vi "InGaAs-GaAs QDSL-111221a.vi"() -> ()   [LabVIEW 2011]
panel:
  out "step number  5":i32
  in  "Number of \nGrowth Steps 5":i32=10
  out "step number  4":i32
  in  "Number of \nGrowth Steps 4":i32=10
  out "step number  3":i32
  in  "Number of \nGrowth Steps 3":i32=10
  out "step number  2":i32
  in  "Number of \nGrowth Steps 2":i32=10
  in  "Indium Flow 2":dbl=55.0
  in  "Ga Flow 3":dbl=2.0
  in  "Ga Flow 2":dbl=2.41
  in  "Ga Flow 1":dbl=5.49
  in  "Indium Flow":dbl=44.0
  in  "Number of \nGrowth Steps":i32=10
  out "step number":i32
  in  "As_Gas Flow":dbl=3.4
  in  "Manifold H2 Flow":dbl=720.0
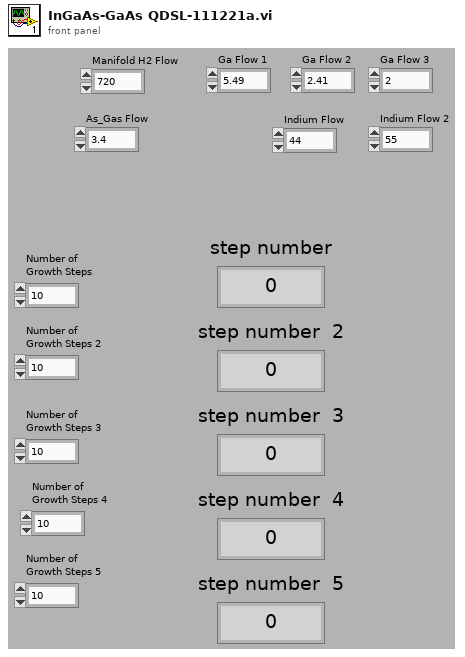
[diagram p1: front panel]
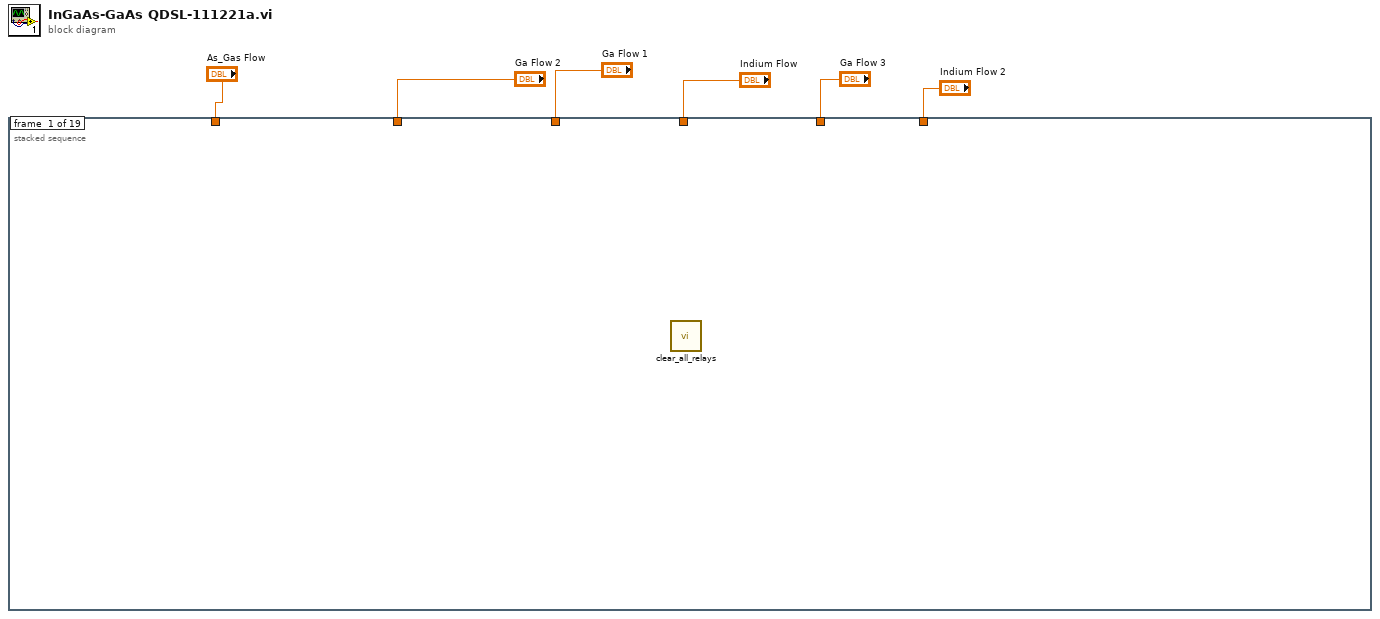
[diagram p0: block diagram]
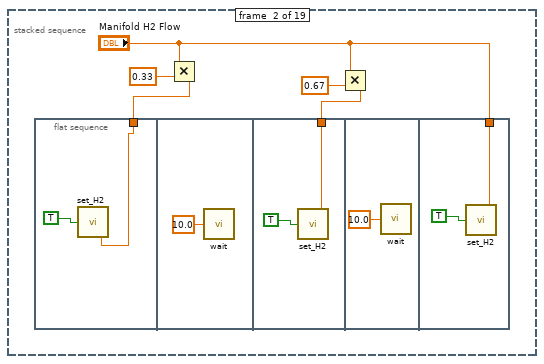
[diagram p2: hidden frame]
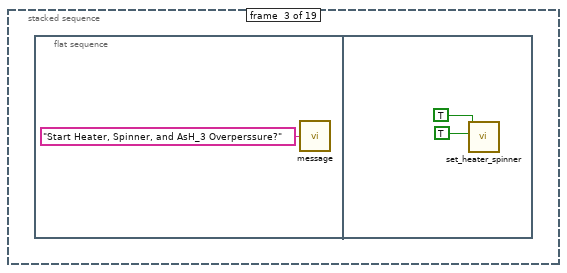
[diagram p3: hidden frame]
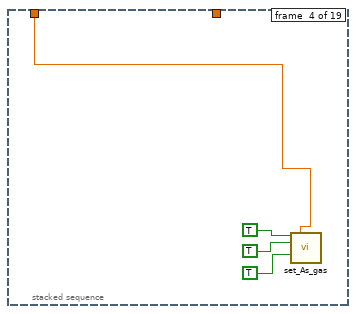
[diagram p4: hidden frame]
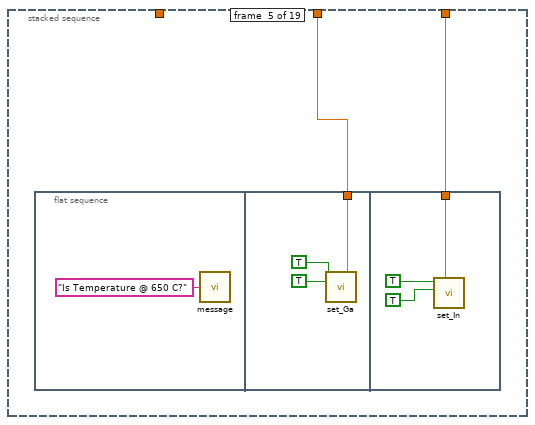
[diagram p5: hidden frame]
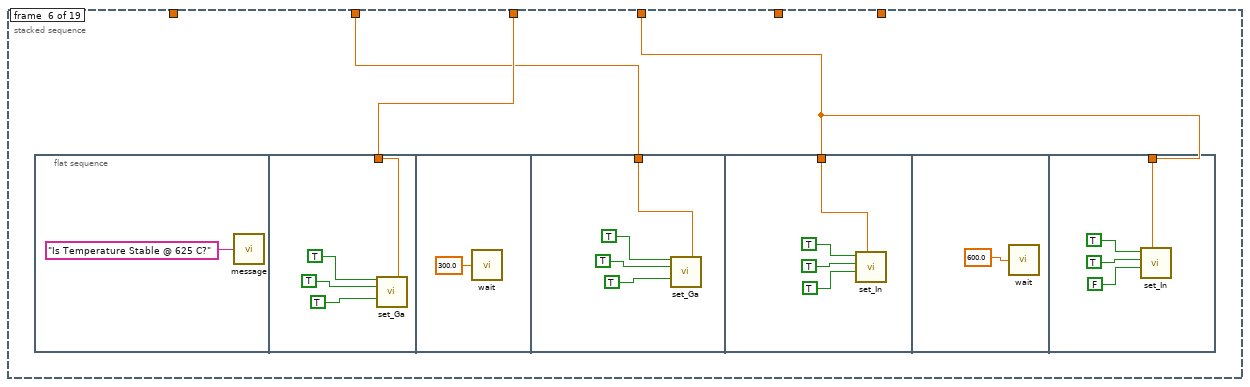
[diagram p6: hidden frame]
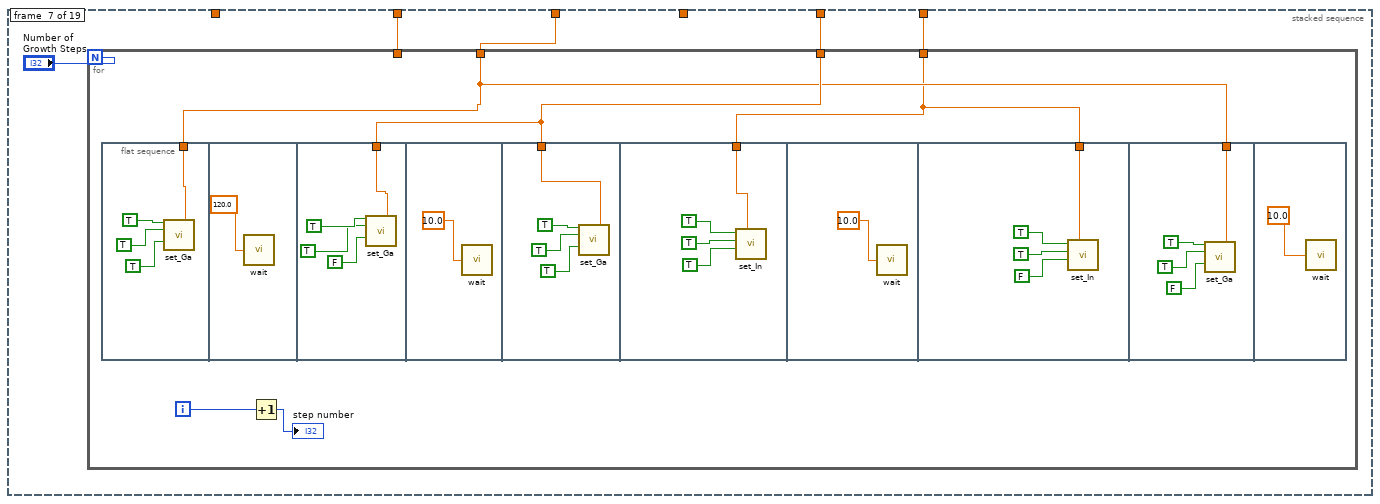
[diagram p7: hidden frame]
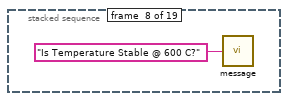
[diagram p8: hidden frame]
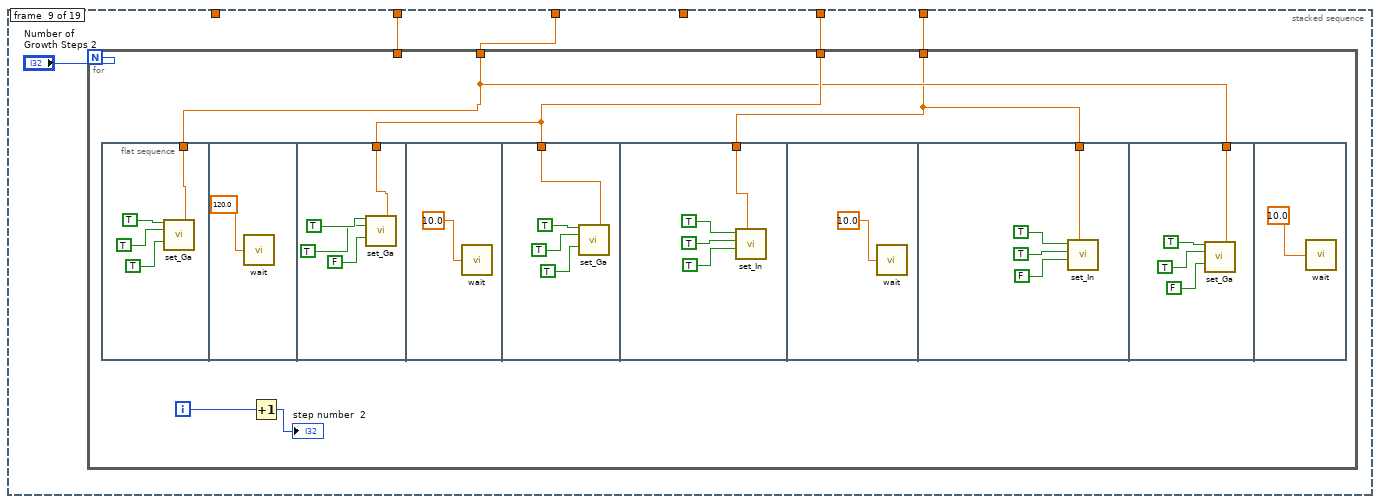
[diagram p9: hidden frame]
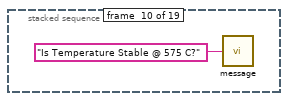
[diagram p10: hidden frame]
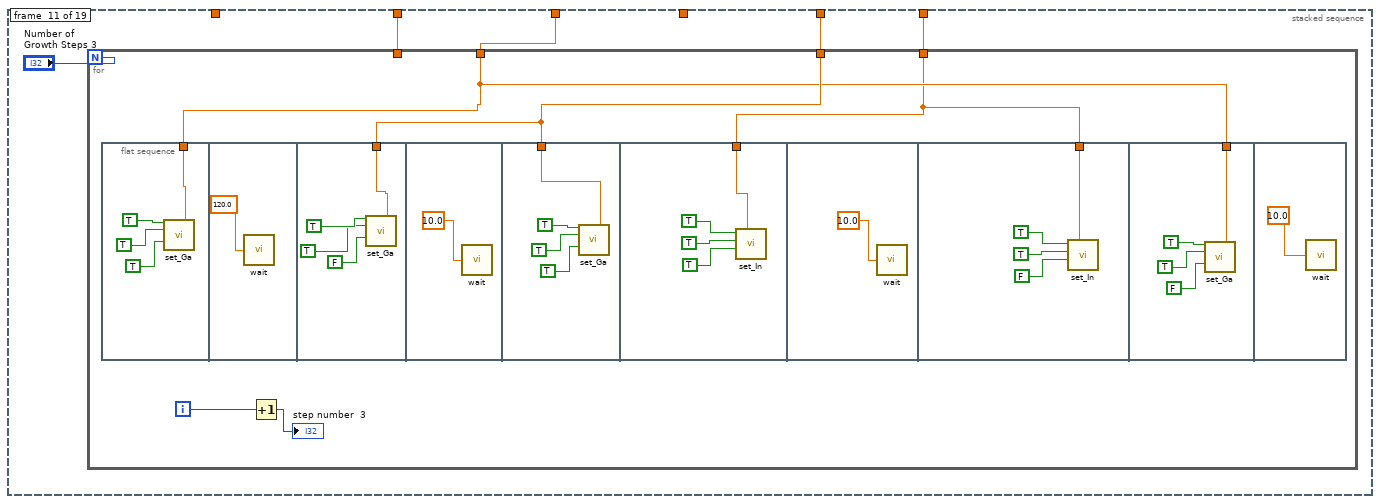
[diagram p11: hidden frame]
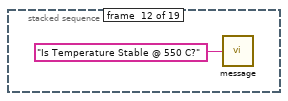
[diagram p12: hidden frame]
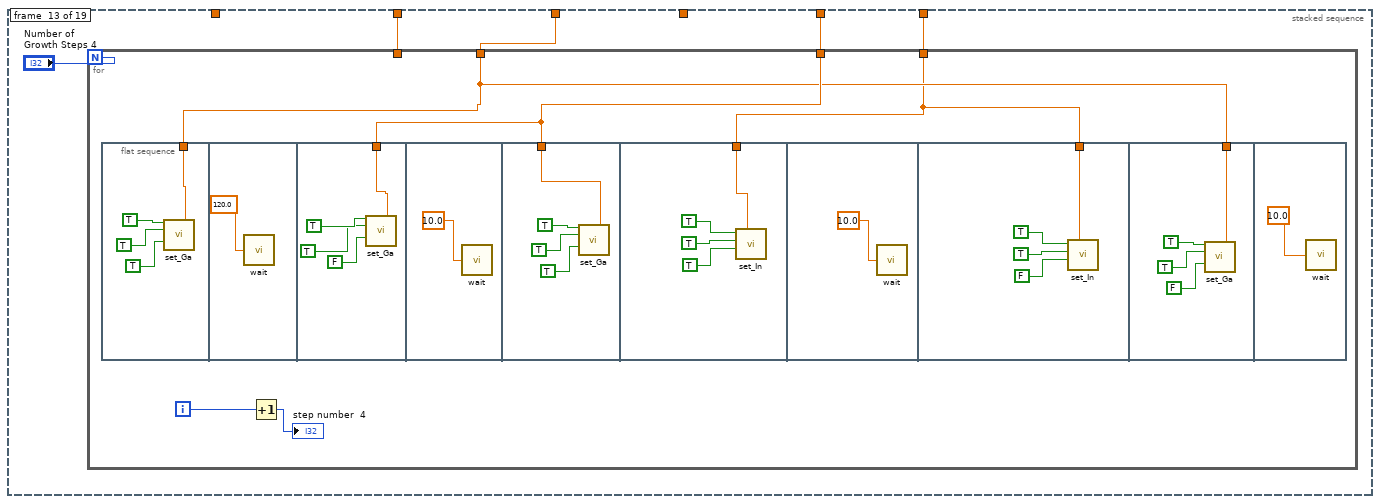
[diagram p13: hidden frame]
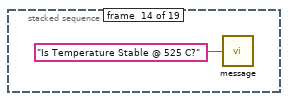
[diagram p14: hidden frame]
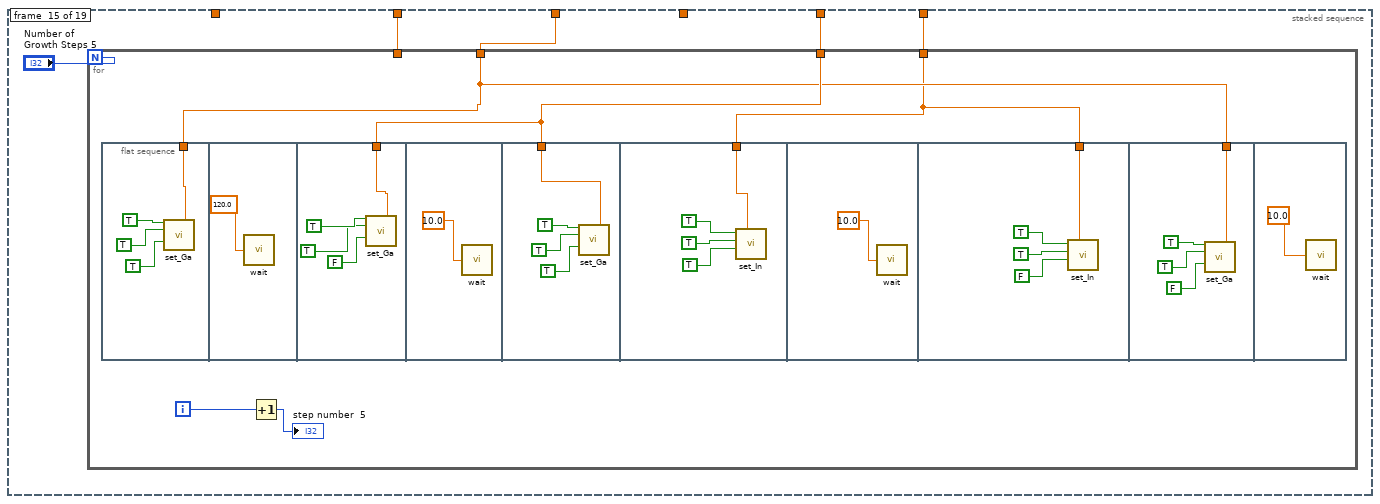
[diagram p15: hidden frame]
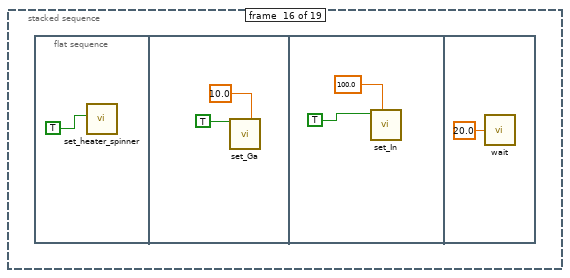
[diagram p16: hidden frame]
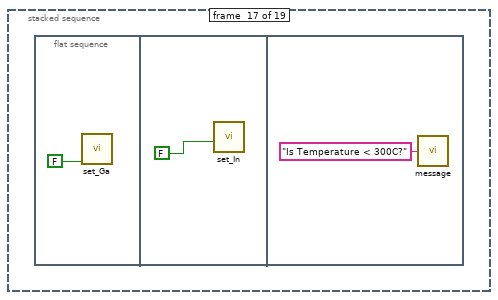
[diagram p17: hidden frame]
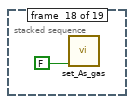
[diagram p18: hidden frame]
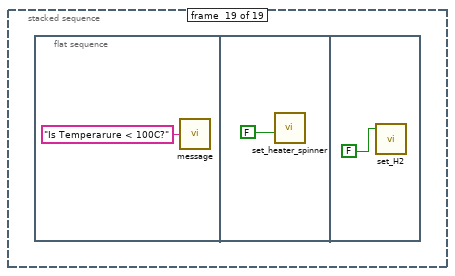
[diagram p19: hidden frame]
diagram:
  n1 = stacked-sequence {
    tunnel: "Ga Flow 1" -> [_ _ _ _ w28 w38 w61 _ w100 _ w139 _ w178 _ w217 _ _ _ _]
    tunnel: "As_Gas Flow" -> [_ _ _ w23 _ _ _ _ _ _ _ _ _ _ _ _ _ _ _]
    tunnel: "Indium Flow" -> [_ _ _ _ w27 w36 _ _ _ _ _ _ _ _ _ _ _ _ _]
    tunnel: "Ga Flow 2" -> [_ _ _ _ _ w37 w60 _ w99 _ w138 _ w177 _ w216 _ _ _ _]
    tunnel: "Ga Flow 3" -> [_ _ _ _ _ _ w59 _ w98 _ w137 _ w176 _ w215 _ _ _ _]
    tunnel: "Indium Flow 2" -> [_ _ _ _ _ _ w58 _ w97 _ w136 _ w175 _ w214 _ _ _ _]
    frame #0 {
      n2 = call "clear_all_relays.vi"() -> ()  [unwired: 2 out]
    }
    frame #1 {
      n3 = flat-sequence {
        tunnel: w11 -> [w12]
        tunnel: w9 -> [w15]
        tunnel: "Manifold H2 Flow" -> [w18]
        frame #0 {
          n4 = call "set_H2.vi"("Manifold H2 Flow"=w12, "H2 Active"=TRUE) -> ()  [unwired: 2 in, 2 out]
        }
        frame #1 {
          n5 = call "wait.vi"("Wait (s)"=10.0) -> ()
        }
        frame #2 {
          n6 = call "set_H2.vi"("Manifold H2 Flow"=w15, "H2 Active"=TRUE) -> ()  [unwired: 2 in, 2 out]
        }
        frame #3 {
          n7 = call "wait.vi"("Wait (s)"=10.0) -> ()
        }
        frame #4 {
          n8 = call "set_H2.vi"("Manifold H2 Flow"=w18, "H2 Active"=TRUE) -> ()  [unwired: 2 in, 2 out]
        }
      }
      n9 = Multiply(x="Manifold H2 Flow", y=0.33) -> (x*y=w11:dbl)
      n10 = Multiply(x="Manifold H2 Flow", y=0.67) -> (x*y=w9:dbl)
    }
    frame #2 {
      n11 = flat-sequence {
        frame #0 {
          n12 = call "message.vi"("message"="Start Heater, Spinner, and AsH_3 Overperssure?") -> ()
        }
        frame #1 {
          n13 = call "set_heater_spinner.vi"("Spinner"=TRUE, "Heater"=TRUE) -> ()  [unwired: 1 in, 7 out]
        }
      }
    }
    frame #3 {
      n14 = call "set_As_gas.vi"("As_Gas Active"=TRUE, "As_Gas Flow"=w23, "As_Gas In"=TRUE, "As_Gas Run"=TRUE) -> ()  [unwired: 2 in, 10 out]
    }
    frame #4 {
      n15 = flat-sequence {
        tunnel: w28 -> [w30]
        tunnel: w27 -> [w33]
        frame #0 {
          n16 = call "message.vi"("message"="Is Temperature @ 650 C?") -> ()
        }
        frame #1 {
          n17 = call "set_Ga.vi"("Ga Active"=TRUE, "Ga Flow 1"=w30, "Ga Bubbler"=TRUE) -> ()  [unwired: 5 in, 8 out]
        }
        frame #2 {
          n18 = call "set_In.vi"("Indium Flow"=w33, "In Bubbler"=TRUE ("Ga Bubbler"), "In Active"=TRUE ("Ga Active")) -> ()  [unwired: 2 in, 5 out]
        }
      }
    }
    frame #5 {
      n19 = flat-sequence {
        tunnel: w38 -> [w40]
        tunnel: w37 -> [w45]
        tunnel: w36 -> [w49]
        tunnel: w36 -> [w54]
        frame #0 {
          n20 = call "message.vi"("message"="Is Temperature Stable @ 625 C?") -> ()
        }
        frame #1 {
          n21 = call "set_Ga.vi"("Ga Active"=TRUE ("P_Gas Active"), "Ga Flow 1"=w40, "Ga Bubbler"=TRUE ("P_Gas In"), "Ga Run"=TRUE ("P_Gas Run")) -> ()  [unwired: 4 in, 8 out]
        }
        frame #2 {
          n22 = call "wait.vi"("Wait (s)"=300.0) -> ()
        }
        frame #3 {
          n23 = call "set_Ga.vi"("Ga Active"=TRUE ("P_Gas Active"), "Ga Flow 1"=w45, "Ga Bubbler"=TRUE ("P_Gas In"), "Ga Run"=TRUE ("P_Gas Run")) -> ()  [unwired: 4 in, 8 out]
        }
        frame #4 {
          n24 = call "set_In.vi"("Indium Flow"=w49, "In Run"=TRUE ("P_Gas Run"), "In Bubbler"=TRUE ("P_Gas In"), "In Active"=TRUE ("P_Gas Active")) -> ()  [unwired: 1 in, 5 out]
        }
        frame #5 {
          n25 = call "wait.vi"("Wait (s)"=600.0) -> ()
        }
        frame #6 {
          n26 = call "set_In.vi"("Indium Flow"=w54, "In Run"=FALSE ("P_Gas Run"), "In Bubbler"=TRUE ("P_Gas In"), "In Active"=TRUE ("P_Gas Active")) -> ()  [unwired: 1 in, 5 out]
        }
      }
    }
    frame #6 {
      n27 = for {
        N: "Number of \nGrowth Steps" -> [_]
        tunnel: w61 -> [w64]
        tunnel: w60 -> [_]
        tunnel: w59 -> [w65]
        tunnel: w58 -> [w63]
        i -> [w66]
        n28 = flat-sequence {
          tunnel: w64 -> [w68]
          tunnel: w65 -> [w73]
          tunnel: w65 -> [w78]
          tunnel: w63 -> [w82]
          tunnel: w63 -> [w87]
          tunnel: w64 -> [w91]
          frame #0 {
            n29 = call "set_Ga.vi"("Ga Active"=TRUE ("P_Gas Active"), "Ga Flow 1"=w68, "Ga Bubbler"=TRUE ("P_Gas In"), "Ga Run"=TRUE ("P_Gas Run")) -> ()  [unwired: 4 in, 8 out]
          }
          frame #1 {
            n30 = call "wait.vi"("Wait (s)"=120.0) -> ()
          }
          frame #2 {
            n31 = call "set_Ga.vi"("Ga Active"=TRUE ("P_Gas Active"), "Ga Flow 1"=w73, "Ga Bubbler"=TRUE ("P_Gas In"), "Ga Run"=FALSE ("P_Gas Run")) -> ()  [unwired: 4 in, 8 out]
          }
          frame #3 {
            n32 = call "wait.vi"("Wait (s)"=10.0) -> ()
          }
          frame #4 {
            n33 = call "set_Ga.vi"("Ga Active"=TRUE ("P_Gas Active"), "Ga Flow 1"=w78, "Ga Bubbler"=TRUE ("P_Gas In"), "Ga Run"=TRUE ("P_Gas Run")) -> ()  [unwired: 4 in, 8 out]
          }
          frame #5 {
            n34 = call "set_In.vi"("Indium Flow"=w82, "In Run"=TRUE ("P_Gas Run"), "In Bubbler"=TRUE ("P_Gas In"), "In Active"=TRUE ("P_Gas Active")) -> ()  [unwired: 1 in, 5 out]
          }
          frame #6 {
            n35 = call "wait.vi"("Wait (s)"=10.0) -> ()
          }
          frame #7 {
            n36 = call "set_In.vi"("Indium Flow"=w87, "In Run"=FALSE ("P_Gas Run"), "In Bubbler"=TRUE ("P_Gas In"), "In Active"=TRUE ("P_Gas Active")) -> ()  [unwired: 1 in, 5 out]
          }
          frame #8 {
            n37 = call "set_Ga.vi"("Ga Active"=TRUE ("P_Gas Active"), "Ga Flow 1"=w91, "Ga Bubbler"=TRUE ("P_Gas In"), "Ga Run"=FALSE ("P_Gas Run")) -> ()  [unwired: 4 in, 8 out]
          }
          frame #9 {
            n38 = call "wait.vi"("Wait (s)"=10.0) -> ()
          }
        }
        n39 = Increment(x=w66) -> (x+1=→"step number":i32)
      }
    }
    frame #7 {
      n40 = call "message.vi"("message"="Is Temperature Stable @ 600 C?") -> ()
    }
    frame #8 {
      n41 = for {
        N: "Number of \nGrowth Steps 2" -> [_]
        tunnel: w100 -> [w103]
        tunnel: w99 -> [_]
        tunnel: w98 -> [w104]
        tunnel: w97 -> [w102]
        i -> [w105]
        n42 = flat-sequence {
          tunnel: w103 -> [w107]
          tunnel: w104 -> [w112]
          tunnel: w104 -> [w117]
          tunnel: w102 -> [w121]
          tunnel: w102 -> [w126]
          tunnel: w103 -> [w130]
          frame #0 {
            n43 = call "set_Ga.vi"("Ga Active"=TRUE ("P_Gas Active"), "Ga Flow 1"=w107, "Ga Bubbler"=TRUE ("P_Gas In"), "Ga Run"=TRUE ("P_Gas Run")) -> ()  [unwired: 4 in, 8 out]
          }
          frame #1 {
            n44 = call "wait.vi"("Wait (s)"=120.0) -> ()
          }
          frame #2 {
            n45 = call "set_Ga.vi"("Ga Active"=TRUE ("P_Gas Active"), "Ga Flow 1"=w112, "Ga Bubbler"=TRUE ("P_Gas In"), "Ga Run"=FALSE ("P_Gas Run")) -> ()  [unwired: 4 in, 8 out]
          }
          frame #3 {
            n46 = call "wait.vi"("Wait (s)"=10.0) -> ()
          }
          frame #4 {
            n47 = call "set_Ga.vi"("Ga Active"=TRUE ("P_Gas Active"), "Ga Flow 1"=w117, "Ga Bubbler"=TRUE ("P_Gas In"), "Ga Run"=TRUE ("P_Gas Run")) -> ()  [unwired: 4 in, 8 out]
          }
          frame #5 {
            n48 = call "set_In.vi"("Indium Flow"=w121, "In Run"=TRUE ("P_Gas Run"), "In Bubbler"=TRUE ("P_Gas In"), "In Active"=TRUE ("P_Gas Active")) -> ()  [unwired: 1 in, 5 out]
          }
          frame #6 {
            n49 = call "wait.vi"("Wait (s)"=10.0) -> ()
          }
          frame #7 {
            n50 = call "set_In.vi"("Indium Flow"=w126, "In Run"=FALSE ("P_Gas Run"), "In Bubbler"=TRUE ("P_Gas In"), "In Active"=TRUE ("P_Gas Active")) -> ()  [unwired: 1 in, 5 out]
          }
          frame #8 {
            n51 = call "set_Ga.vi"("Ga Active"=TRUE ("P_Gas Active"), "Ga Flow 1"=w130, "Ga Bubbler"=TRUE ("P_Gas In"), "Ga Run"=FALSE ("P_Gas Run")) -> ()  [unwired: 4 in, 8 out]
          }
          frame #9 {
            n52 = call "wait.vi"("Wait (s)"=10.0) -> ()
          }
        }
        n53 = Increment(x=w105) -> (x+1=→"step number  2":i32)
      }
    }
    frame #9 {
      n54 = call "message.vi"("message"="Is Temperature Stable @ 575 C?") -> ()
    }
    frame #10 {
      n55 = for {
        N: "Number of \nGrowth Steps 3" -> [_]
        tunnel: w139 -> [w142]
        tunnel: w138 -> [_]
        tunnel: w137 -> [w143]
        tunnel: w136 -> [w141]
        i -> [w144]
        n56 = flat-sequence {
          tunnel: w142 -> [w146]
          tunnel: w143 -> [w151]
          tunnel: w143 -> [w156]
          tunnel: w141 -> [w160]
          tunnel: w141 -> [w165]
          tunnel: w142 -> [w169]
          frame #0 {
            n57 = call "set_Ga.vi"("Ga Active"=TRUE ("P_Gas Active"), "Ga Flow 1"=w146, "Ga Bubbler"=TRUE ("P_Gas In"), "Ga Run"=TRUE ("P_Gas Run")) -> ()  [unwired: 4 in, 8 out]
          }
          frame #1 {
            n58 = call "wait.vi"("Wait (s)"=120.0) -> ()
          }
          frame #2 {
            n59 = call "set_Ga.vi"("Ga Active"=TRUE ("P_Gas Active"), "Ga Flow 1"=w151, "Ga Bubbler"=TRUE ("P_Gas In"), "Ga Run"=FALSE ("P_Gas Run")) -> ()  [unwired: 4 in, 8 out]
          }
          frame #3 {
            n60 = call "wait.vi"("Wait (s)"=10.0) -> ()
          }
          frame #4 {
            n61 = call "set_Ga.vi"("Ga Active"=TRUE ("P_Gas Active"), "Ga Flow 1"=w156, "Ga Bubbler"=TRUE ("P_Gas In"), "Ga Run"=TRUE ("P_Gas Run")) -> ()  [unwired: 4 in, 8 out]
          }
          frame #5 {
            n62 = call "set_In.vi"("Indium Flow"=w160, "In Run"=TRUE ("P_Gas Run"), "In Bubbler"=TRUE ("P_Gas In"), "In Active"=TRUE ("P_Gas Active")) -> ()  [unwired: 1 in, 5 out]
          }
          frame #6 {
            n63 = call "wait.vi"("Wait (s)"=10.0) -> ()
          }
          frame #7 {
            n64 = call "set_In.vi"("Indium Flow"=w165, "In Run"=FALSE ("P_Gas Run"), "In Bubbler"=TRUE ("P_Gas In"), "In Active"=TRUE ("P_Gas Active")) -> ()  [unwired: 1 in, 5 out]
          }
          frame #8 {
            n65 = call "set_Ga.vi"("Ga Active"=TRUE ("P_Gas Active"), "Ga Flow 1"=w169, "Ga Bubbler"=TRUE ("P_Gas In"), "Ga Run"=FALSE ("P_Gas Run")) -> ()  [unwired: 4 in, 8 out]
          }
          frame #9 {
            n66 = call "wait.vi"("Wait (s)"=10.0) -> ()
          }
        }
        n67 = Increment(x=w144) -> (x+1=→"step number  3":i32)
      }
    }
    frame #11 {
      n68 = call "message.vi"("message"="Is Temperature Stable @ 550 C?") -> ()
    }
    frame #12 {
      n69 = for {
        N: "Number of \nGrowth Steps 4" -> [_]
        tunnel: w178 -> [w181]
        tunnel: w177 -> [_]
        tunnel: w176 -> [w182]
        tunnel: w175 -> [w180]
        i -> [w183]
        n70 = flat-sequence {
          tunnel: w181 -> [w185]
          tunnel: w182 -> [w190]
          tunnel: w182 -> [w195]
          tunnel: w180 -> [w199]
          tunnel: w180 -> [w204]
          tunnel: w181 -> [w208]
          frame #0 {
            n71 = call "set_Ga.vi"("Ga Active"=TRUE ("P_Gas Active"), "Ga Flow 1"=w185, "Ga Bubbler"=TRUE ("P_Gas In"), "Ga Run"=TRUE ("P_Gas Run")) -> ()  [unwired: 4 in, 8 out]
          }
          frame #1 {
            n72 = call "wait.vi"("Wait (s)"=120.0) -> ()
          }
          frame #2 {
            n73 = call "set_Ga.vi"("Ga Active"=TRUE ("P_Gas Active"), "Ga Flow 1"=w190, "Ga Bubbler"=TRUE ("P_Gas In"), "Ga Run"=FALSE ("P_Gas Run")) -> ()  [unwired: 4 in, 8 out]
          }
          frame #3 {
            n74 = call "wait.vi"("Wait (s)"=10.0) -> ()
          }
          frame #4 {
            n75 = call "set_Ga.vi"("Ga Active"=TRUE ("P_Gas Active"), "Ga Flow 1"=w195, "Ga Bubbler"=TRUE ("P_Gas In"), "Ga Run"=TRUE ("P_Gas Run")) -> ()  [unwired: 4 in, 8 out]
          }
          frame #5 {
            n76 = call "set_In.vi"("Indium Flow"=w199, "In Run"=TRUE ("P_Gas Run"), "In Bubbler"=TRUE ("P_Gas In"), "In Active"=TRUE ("P_Gas Active")) -> ()  [unwired: 1 in, 5 out]
          }
          frame #6 {
            n77 = call "wait.vi"("Wait (s)"=10.0) -> ()
          }
          frame #7 {
            n78 = call "set_In.vi"("Indium Flow"=w204, "In Run"=FALSE ("P_Gas Run"), "In Bubbler"=TRUE ("P_Gas In"), "In Active"=TRUE ("P_Gas Active")) -> ()  [unwired: 1 in, 5 out]
          }
          frame #8 {
            n79 = call "set_Ga.vi"("Ga Active"=TRUE ("P_Gas Active"), "Ga Flow 1"=w208, "Ga Bubbler"=TRUE ("P_Gas In"), "Ga Run"=FALSE ("P_Gas Run")) -> ()  [unwired: 4 in, 8 out]
          }
          frame #9 {
            n80 = call "wait.vi"("Wait (s)"=10.0) -> ()
          }
        }
        n81 = Increment(x=w183) -> (x+1=→"step number  4":i32)
      }
    }
    frame #13 {
      n82 = call "message.vi"("message"="Is Temperature Stable @ 525 C?") -> ()
    }
    frame #14 {
      n83 = for {
        N: "Number of \nGrowth Steps 5" -> [_]
        tunnel: w217 -> [w220]
        tunnel: w216 -> [_]
        tunnel: w215 -> [w221]
        tunnel: w214 -> [w219]
        i -> [w222]
        n84 = flat-sequence {
          tunnel: w220 -> [w224]
          tunnel: w221 -> [w229]
          tunnel: w221 -> [w234]
          tunnel: w219 -> [w238]
          tunnel: w219 -> [w243]
          tunnel: w220 -> [w247]
          frame #0 {
            n85 = call "set_Ga.vi"("Ga Active"=TRUE ("P_Gas Active"), "Ga Flow 1"=w224, "Ga Bubbler"=TRUE ("P_Gas In"), "Ga Run"=TRUE ("P_Gas Run")) -> ()  [unwired: 4 in, 8 out]
          }
          frame #1 {
            n86 = call "wait.vi"("Wait (s)"=120.0) -> ()
          }
          frame #2 {
            n87 = call "set_Ga.vi"("Ga Active"=TRUE ("P_Gas Active"), "Ga Flow 1"=w229, "Ga Bubbler"=TRUE ("P_Gas In"), "Ga Run"=FALSE ("P_Gas Run")) -> ()  [unwired: 4 in, 8 out]
          }
          frame #3 {
            n88 = call "wait.vi"("Wait (s)"=10.0) -> ()
          }
          frame #4 {
            n89 = call "set_Ga.vi"("Ga Active"=TRUE ("P_Gas Active"), "Ga Flow 1"=w234, "Ga Bubbler"=TRUE ("P_Gas In"), "Ga Run"=TRUE ("P_Gas Run")) -> ()  [unwired: 4 in, 8 out]
          }
          frame #5 {
            n90 = call "set_In.vi"("Indium Flow"=w238, "In Run"=TRUE ("P_Gas Run"), "In Bubbler"=TRUE ("P_Gas In"), "In Active"=TRUE ("P_Gas Active")) -> ()  [unwired: 1 in, 5 out]
          }
          frame #6 {
            n91 = call "wait.vi"("Wait (s)"=10.0) -> ()
          }
          frame #7 {
            n92 = call "set_In.vi"("Indium Flow"=w243, "In Run"=FALSE ("P_Gas Run"), "In Bubbler"=TRUE ("P_Gas In"), "In Active"=TRUE ("P_Gas Active")) -> ()  [unwired: 1 in, 5 out]
          }
          frame #8 {
            n93 = call "set_Ga.vi"("Ga Active"=TRUE ("P_Gas Active"), "Ga Flow 1"=w247, "Ga Bubbler"=TRUE ("P_Gas In"), "Ga Run"=FALSE ("P_Gas Run")) -> ()  [unwired: 4 in, 8 out]
          }
          frame #9 {
            n94 = call "wait.vi"("Wait (s)"=10.0) -> ()
          }
        }
        n95 = Increment(x=w222) -> (x+1=→"step number  5":i32)
      }
    }
    frame #15 {
      n96 = flat-sequence {
        frame #0 {
          n97 = call "set_heater_spinner.vi"("Spinner"=TRUE ("Ga Active")) -> ()  [unwired: 2 in, 7 out]
        }
        frame #1 {
          n98 = call "set_Ga.vi"("Ga Active"=TRUE, "Ga Flow 1"=10.0) -> ()  [unwired: 6 in, 8 out]
        }
        frame #2 {
          n99 = call "set_In.vi"("Indium Flow"=100.0 ("Aluminum Flow"), "In Active"=TRUE ("Ga Active")) -> ()  [unwired: 3 in, 5 out]
        }
        frame #3 {
          n100 = call "wait.vi"("Wait (s)"=20.0) -> ()
        }
      }
    }
    frame #16 {
      n101 = flat-sequence {
        frame #0 {
          n102 = call "set_Ga.vi"("Ga Remote"=FALSE) -> ()  [unwired: 7 in, 8 out]
        }
        frame #1 {
          n103 = call "set_In.vi"("In Run"=FALSE ("Ga Remote")) -> ()  [unwired: 4 in, 5 out]
        }
        frame #2 {
          n104 = call "message.vi"("message"="Is Temperature < 300C?") -> ()
        }
      }
    }
    frame #17 {
      n105 = call "set_As_gas.vi"("As_Gas Remote"=FALSE) -> ()  [unwired: 5 in, 10 out]
    }
    frame #18 {
      n106 = flat-sequence {
        frame #0 {
          n107 = call "message.vi"("message"="Is Temperarure < 100C?") -> ()
        }
        frame #1 {
          n108 = call "set_heater_spinner.vi"("Heater/Spinner Remote"=FALSE) -> ()  [unwired: 2 in, 7 out]
        }
        frame #2 {
          n109 = call "set_H2.vi"("H2N2 Remote"=FALSE) -> ()  [unwired: 3 in, 2 out]
        }
      }
    }
  }
